vi "CONTROL CAN Write data.vi"(8 "error in (no error)":errorcluster, 10 "data":dbl[](array[numeric]) format="%.2f") -> (0 "error out":errorcluster)   [LabVIEW 2018]
uses:
  Application/Common VIs/Read File Data.ctl
  <vilib>/xnet/xnet.llb/XNET Create Session (Signal Input Single-point).vi
  <vilib>/xnet/xnet.llb/XNET Write (Signal Single-point).vi
panel:
  in  "stop":bool
  out "session out 2":refnum<k21>
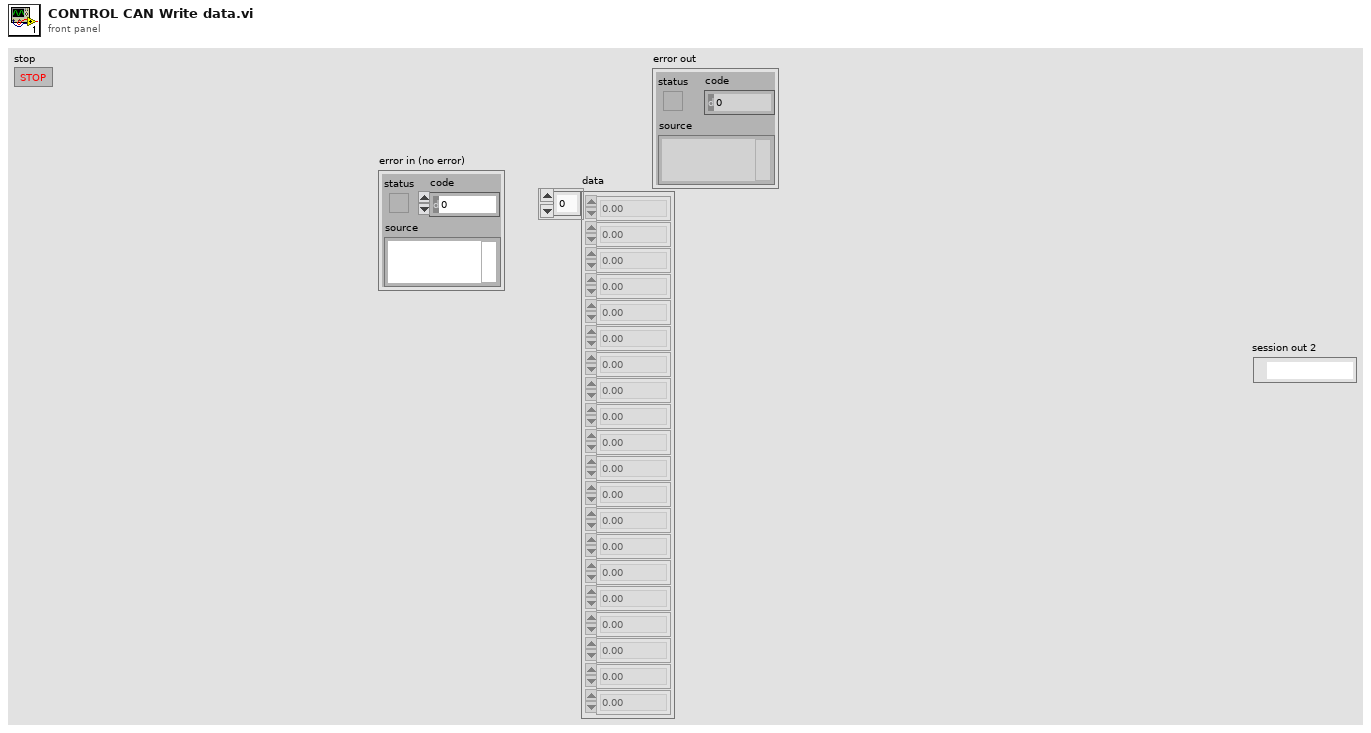
[diagram p1: front panel]
types:
  T1 = typedef "Read File Data.ctl" = enum16{"Get Data", "Set Data"}
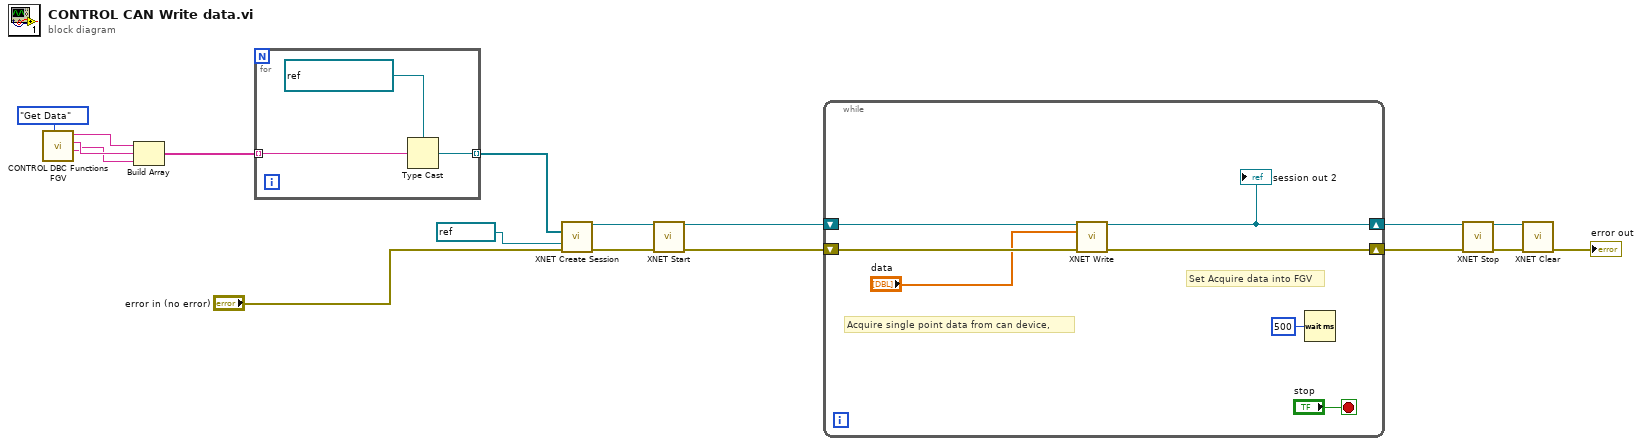
[diagram p0: block diagram]
diagram:
  n1 = call "CONTROL DBC Functions FGV.vi"("Enum"=Read_File_Data."Get Data") -> ("PADDLE OUT"=w2:string, "TORQUE OUT"=w3:string, "SPEED OUT"=w4:string)  [unwired: 7 in, 1 out]
  n2 = Build Array(w4, w3, w2) -> (w1:string[])
  n3 = for {
    tunnel: [w19] -> w6 mode=indexing
    tunnel: w1 -> [w18] mode=indexing
    n4 = Type Cast(type=refnum<k21> "EngineOilPrLamp\nTEST" ("XNET Signal"), x=w18) -> (*(type *) &x=w19:refnum<k21>)
  }
  n5 = call-poly <vilib>:"XNET Create Session.vi"("signal list"=w6, "interface"=refnum<k21> "CAN1" ("Select Interface"), "error in (no error)"="error in (no error)") -> ("session out"=w15:refnum<k21>, "error out"=w16:errorcluster)  [unwired: 11 out]
  n6 = call <vilib>:"XNET Start.vi"("session in"=w15, "error in (no error)"=w16) -> ("session out"=w13:refnum<k21>, "error out"=w12:errorcluster)  [unwired: 12 in]
  n7 = while {
    shift-right: [w25] -> w8
    shift-left: w13 -> [w27]
    shift-right: [w21] -> w9
    shift-left: w12 -> [w26]
    stop <- "stop" stop-if-true
    # "Set Acquire data into FGV"
    # "Acquire single point data from can device,"
    n8 = call-poly <vilib>:"XNET Write.vi"("session in"=w27, "data"="data", "error in (no error)"=w26) -> ("session out"=w25:refnum<k21>, "error out"=w21:errorcluster)  [unwired: 11 in]
    "session out 2" <- w25
    n9 = Wait (ms)(milliseconds to wait=u32 500) -> ()  [unwired: 1 out]
  }
  n10 = call <vilib>:"XNET Stop.vi"("session in"=w8, "error in (no error)"=w9) -> ("session out"=w11:refnum<k21>, "error out"=w10:errorcluster)  [unwired: 12 in]
  n11 = call <vilib>:"XNET Clear.vi"("session in"=w11, "error in (no error)"=w10) -> ("error out"=→"error out":errorcluster)  [unwired: 13 in]
